vi "DMM Read Voltage.vi"(6 "Timeout (5000 milliseconds)":u32=1000, 8 "error in (no error)":errorcluster, 11 "DMM":refnum<visa-resource-name>="COM1") -> (0 "error out":errorcluster, 1 "Voltage":dbl format="%0.8f", 2 "Voltage Data":dbl[](array[numeric]))   [LabVIEW 2015]
uses:
  <instrlib>/Keithley 27XX/Public/Data/Read Multiple Direct.vi
  <instrlib>/Keithley 27XX/Keithley 27XX.lvlib
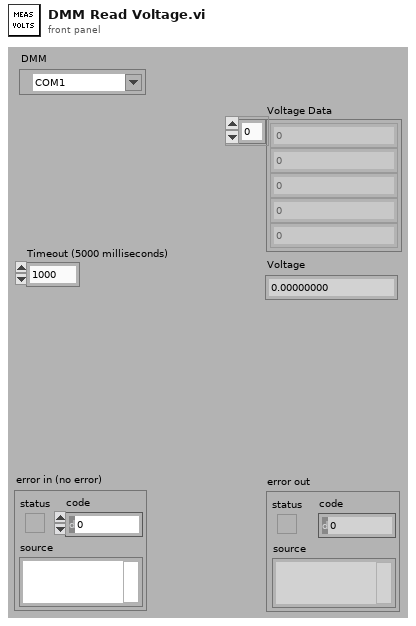
[diagram p1: front panel]
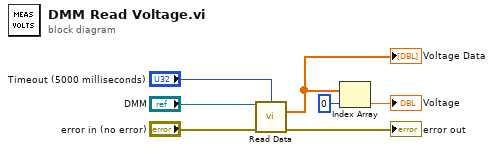
[diagram p0: block diagram]
diagram:
  n1 = call-poly <instrlib>:"Read Data.vi"("VISA resource name"="DMM", "Timeout (30000 milliseconds)"="Timeout (5000 milliseconds)", "error in (no error)"="error in (no error)") -> ("Measurement Data"=w6:dbl[], "error out"=→"error out":errorcluster)  [unwired: 7 in, 4 out]
  "Voltage Data" <- w6
  n2 = Index Array(array=w6, index=0) -> (element=→"Voltage":dbl)
